vi "GetVariableDataResults.vi"(7 "taskId":i32(ring) items=["TLibrary", "T01", "T02", "T03", "T04", "T05", "T06", "T07", "T08", "T09", "T10", "T11", "T12", "T13", "T14", "T15", "T16", "T17", "T18", "T19", "T20", "T21", "T22", "T23", "T24", "T25", "T26", "T27", "T28", "T29", "T30", "T31"], 8 "error in (no error)":errorcluster, 9 "variable name":string, 10 "Data In":refnum<k24>, 11 "controller in":refnum<k24>) -> (0 "error out":errorcluster, 1 "VariableData":dbl[](array[numeric]), 2 "Data Out":refnum<k24>, 3 "controller out":refnum<k24>)   [LabVIEW 2010]
uses:
  c:/aerotech/controller/5.xx.xxx/A3200/pc/labview/2010/bin/Aerotech.A3200.dll
  bin/Aerotech.A3200.dll
  c:/aerotech/controller/5.xx.xxx/A3200/pc/labview/2010/bin/Aerotech.A3200.LabVIEW.dll
  bin/Aerotech.A3200.LabVIEW.dll
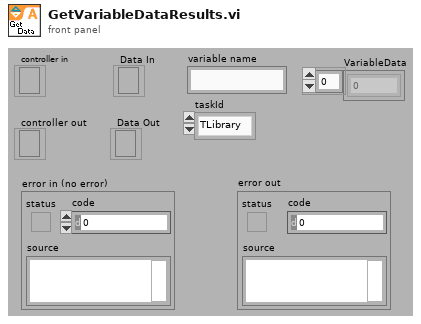
[diagram p1: front panel]
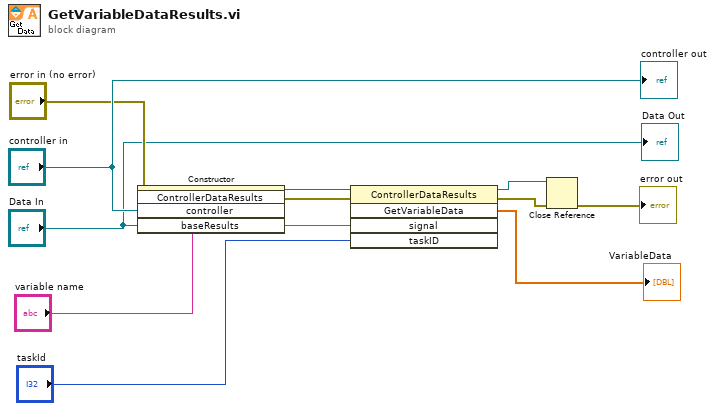
[diagram p0: block diagram]
diagram:
  n1 = constructor class="ControllerDataResults"(error in="error in (no error)", "controller"="controller in", "baseResults"="Data In") -> (reference out=w9:refnum<k24>, error out=w10:errorcluster)  [unwired: 2 in, 3 out]
  n2 = invoke class="ControllerDataResults" method="GetVariableData"(reference=w9, error in=w10, "signal"="variable name", "taskID"="taskId") -> (reference out=w7:refnum<k24>, error out=w8:errorcluster, "GetVariableData"=→"VariableData":dbl[])  [unwired: 1 in, 2 out]
  n3 = Close Reference(reference=w7, error in (no error)=w8) -> (error out=→"error out":errorcluster)
  "controller out" <- "controller in"
  "Data Out" <- "Data In"
